vi "OutputRT.vi"(6 "Bias in":refnum<k21>, 7 "Monitor Task":refnum<k21>, 8 "rate":dbl=1000.0 format="%0.2f", 9 "MessageQueues":T1, 10 "Bias Voltage (mV)":string, 11 "TraceTime":dbl) -> ()   [LabVIEW 2024]
uses:
  MessageQueues.ctl
  <vilib>/httpClient/ClientHandle.ctl
  <vilib>/DAQmx/write.llb/DAQmx Write (Analog DBL 1Chan 1Samp).vi
  <vilib>/DAQmx/configure/timing.llb/DAQmx Timing (Sample Clock).vi
  <vilib>/DAQmx/miscellaneous.llb/DAQmx Fill In Error Info.vi
  <vilib>/httpClient/LabVIEWHTTPClient.lvlib
panel:
  in  "Sampling Rate: 3":dbl=5000.0
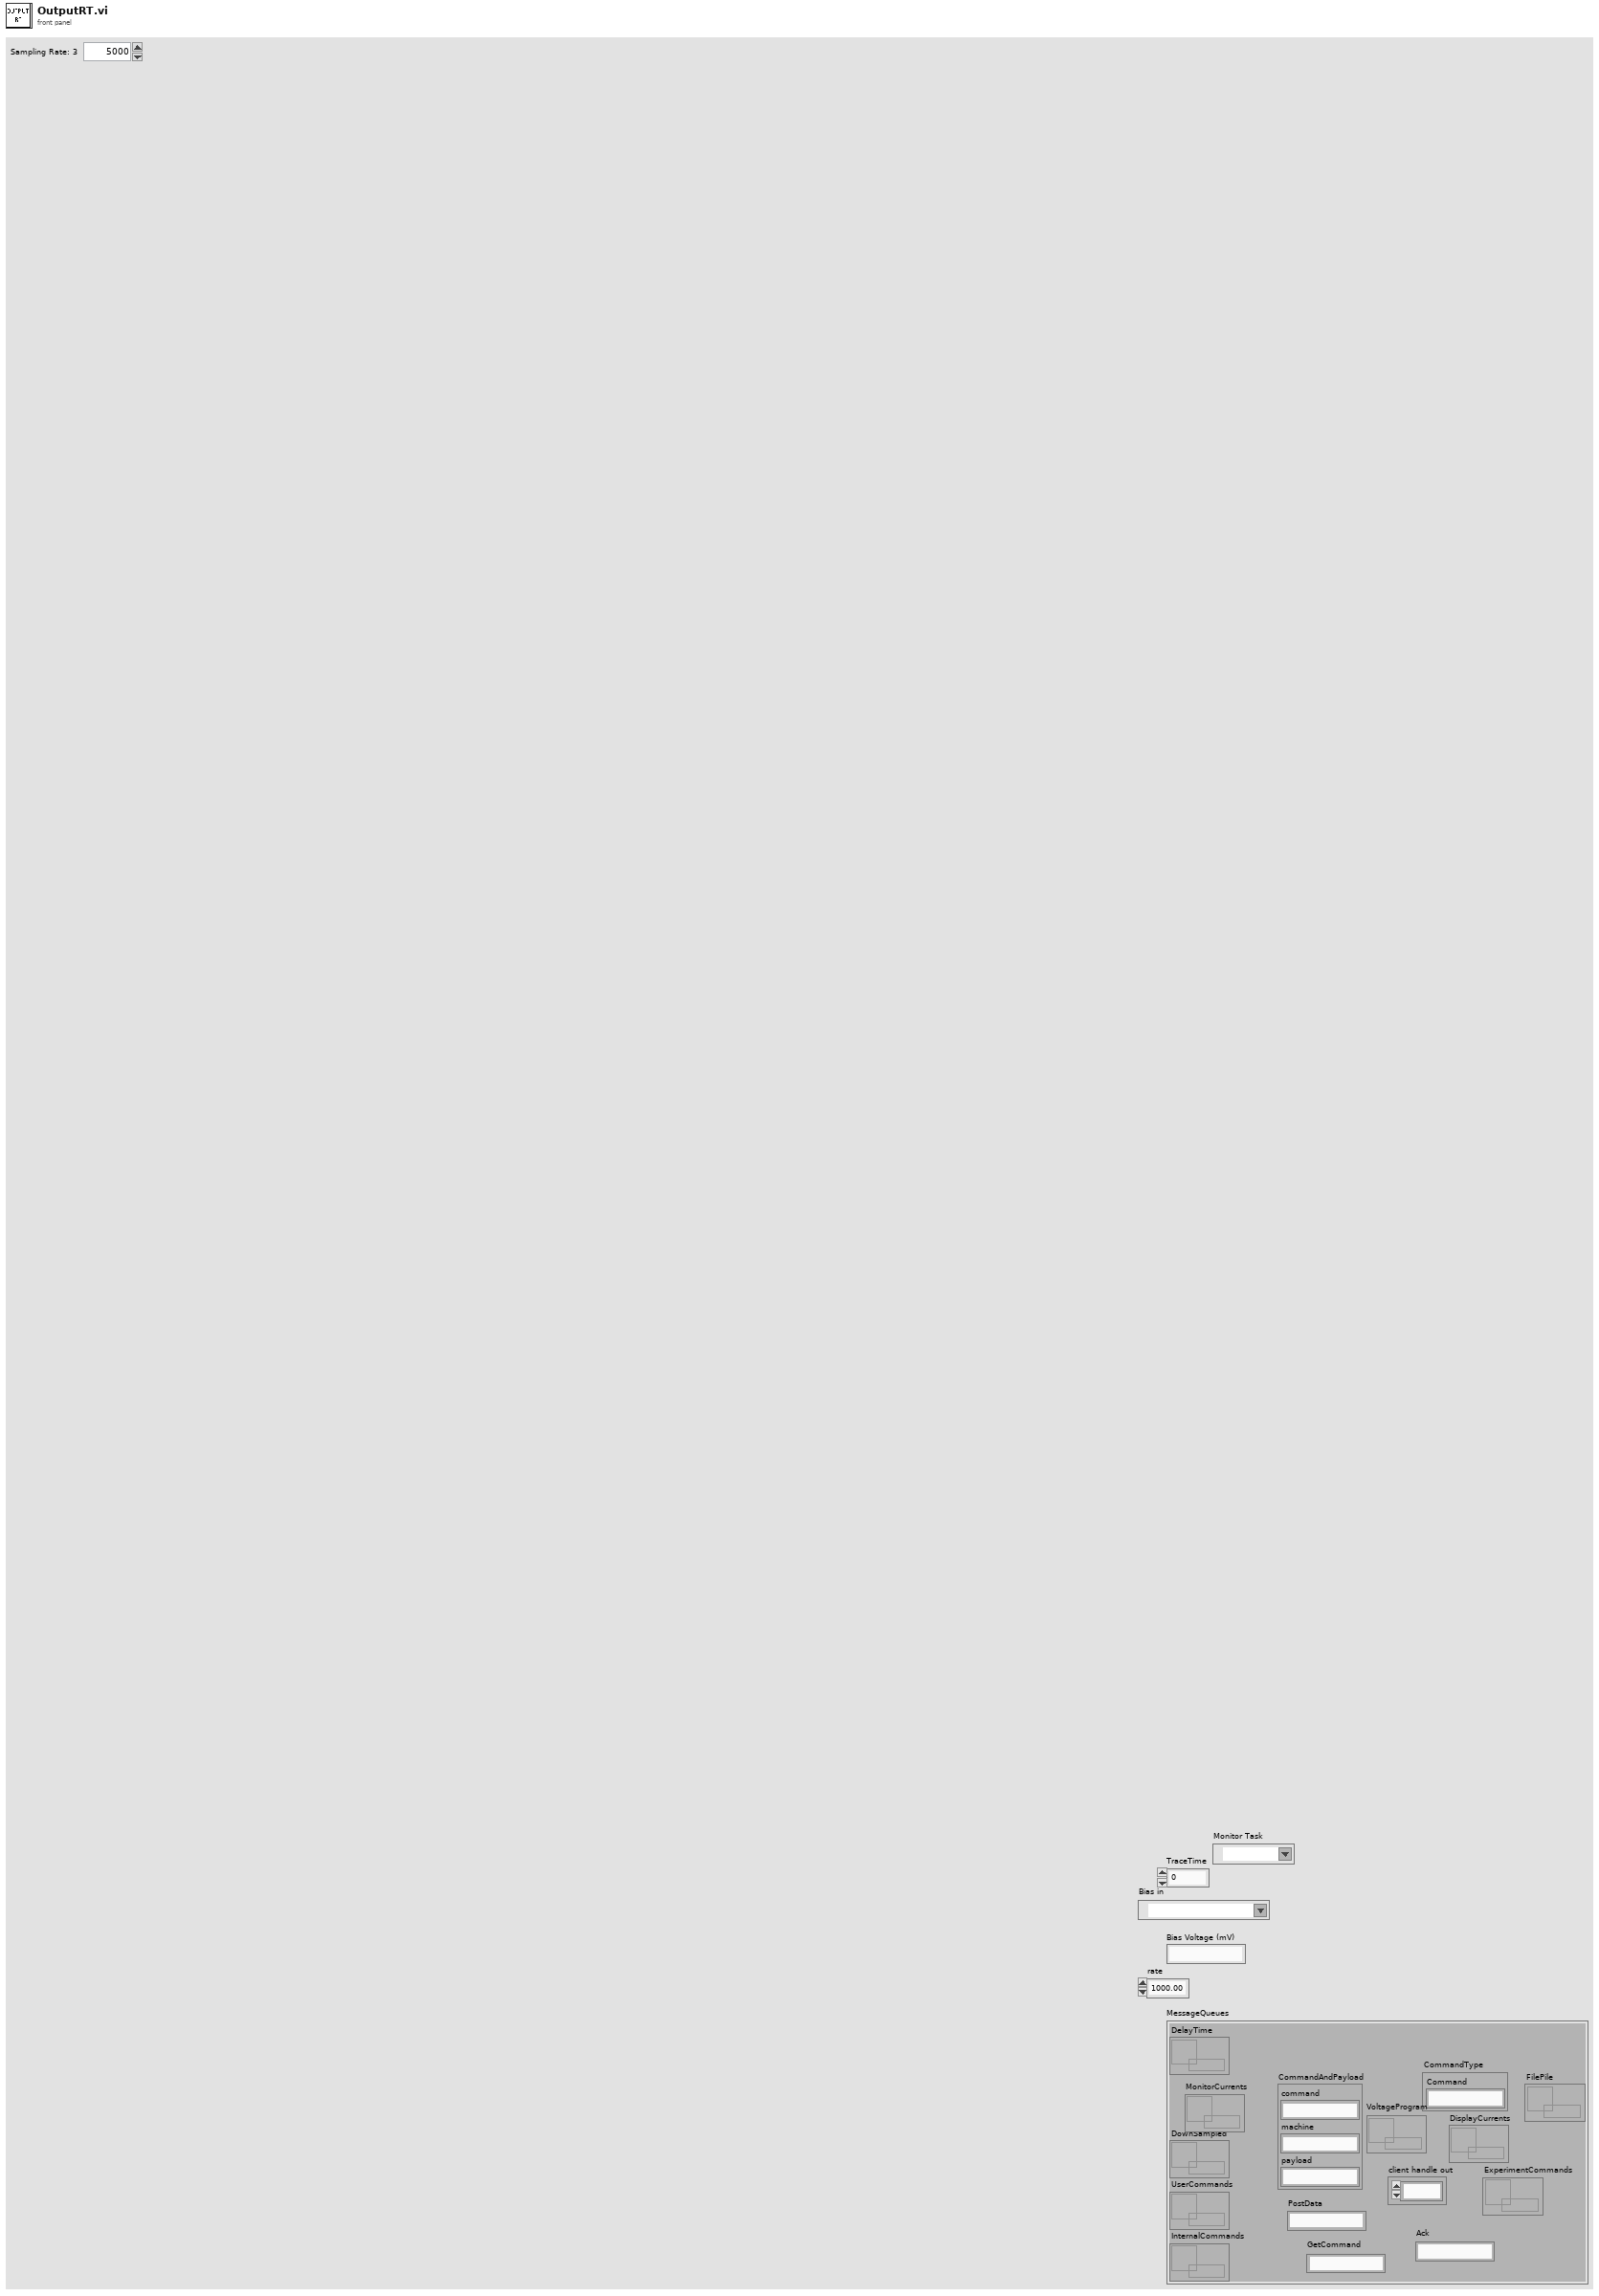
[diagram p1: front panel]
types:
  T1 = typedef "MessageQueues.ctl" = cluster{"DelayTime":refnum<queue>, "DownSampled":refnum<queue>, "UserCommands":refnum<queue>, "InternalCommands":refnum<queue>, "CommandType":cluster{"Command":string}, "CommandAndPayload":cluster{"command":string, "machine":string, "payload":string}, "client handle out":T2, "PostData":string, "GetCommand":string, "Ack":string, "VoltageProgram":refnum<queue>, "ExperimentCommands":refnum<queue>, "DisplayCurrents":refnum<queue>, "MonitorCurrents":refnum<queue>, "FilePile":refnum<queue>}
  T2 = typedef "LabVIEWHTTPClient.lvlib/ClientHandle.ctl" = refnum<k1>
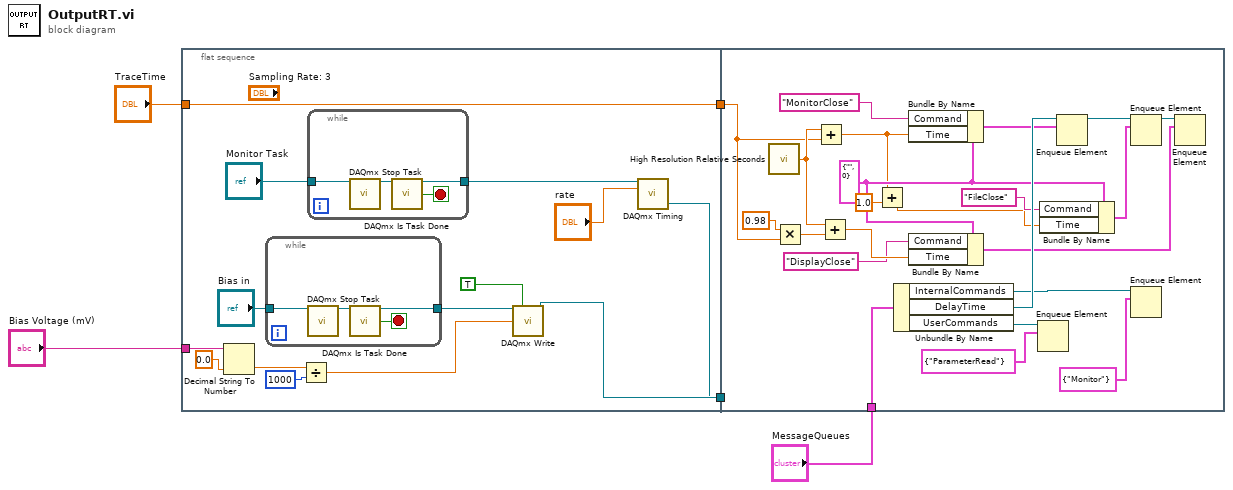
[diagram p0: block diagram]
diagram:
  n1 = flat-sequence {
    tunnel: [w20] -> w6
    tunnel: "TraceTime" -> [w20]
    tunnel: "Bias Voltage (mV)" -> [w18]
    tunnel: [w13] -> w5
    tunnel: [w11] -> w1
    tunnel: w6 -> [w33]
    tunnel: "MessageQueues" -> [w51]
    tunnel: w5 -> [_]
    tunnel: w1 -> [_]
    frame #0 {
      n2 = Decimal String To Number(string=w18, default (0L)=0.0) -> (number=w16:dbl)  [unwired: 1 in, 1 out]
      n3 = while {
        tunnel: "Bias in" -> [w28]
        tunnel: [w26] -> w9
        stop <- w25 stop-if-true
        n4 = call <vilib>:"DAQmx Stop Task.vi"("task/channels in"=w28) -> ("task out"=w27:refnum<k21>)  [unwired: 13 in, 1 out]
        n5 = call <vilib>:"DAQmx Is Task Done.vi"("task/channels in"=w27) -> ("task out"=w26:refnum<k21>, "task done?"=w25:bool)  [unwired: 12 in, 1 out]
      }
      n6 = Divide(x=w16, y=1000) -> (x/y=w15:dbl)
      n7 = while {
        tunnel: "Monitor Task" -> [w24]
        tunnel: [w22] -> w7
        stop <- w21 stop-if-true
        n8 = call <vilib>:"DAQmx Stop Task.vi"("task/channels in"=w24) -> ("task out"=w23:refnum<k21>)  [unwired: 13 in, 1 out]
        n9 = call <vilib>:"DAQmx Is Task Done.vi"("task/channels in"=w23) -> ("task out"=w22:refnum<k21>, "task done?"=w21:bool)  [unwired: 12 in, 1 out]
      }
      n10 = call-poly <vilib>:"DAQmx Write.vi"("task/channels in"=w9, "auto start"=TRUE, "data"=w15) -> ("task out"=w13:refnum<k21>)  [unwired: 10 in, 2 out]
      n11 = call-poly <vilib>:"DAQmx Timing.vi"("task/channels in"=w7, "rate"="rate") -> ("task out"=w11:refnum<k21>)  [unwired: 12 in, 1 out]
    }
    frame #1 {
      w36 = cluster{"Command":string, "Time":i32} {"Command"="", "Time"=0} ("element")
      n12 = call <vilib>:"High Resolution Relative Seconds.vi"() -> ("relative seconds"=w40:dbl)
      n13 = Multiply(x=0.98, y=w33) -> (x*y=w32:dbl)
      n14 = Add(x=w40, y=w33) -> (x+y=w31:dbl)
      n15 = Add(x=w40, y=w32) -> (x+y=w35:dbl)
      n16 = Add(x=w31, y=1.0) -> (x+y=w30:dbl)
      n17 = Unbundle By Name(w51) -> ("InternalCommands"=w45:refnum<queue>, "DelayTime"=w50:refnum<queue>, "UserCommands"=w46:refnum<queue>)
      n18 = Bundle By Name(cluster=w36, "Command"="MonitorClose", "Time"=w31) -> (w49:cluster{"Command":string, "Time":i32})
      n19 = Bundle By Name(cluster=w36, "Command"="DisplayClose", "Time"=w35) -> (w37:cluster{"Command":string, "Time":i32})
      n20 = Enqueue Element(queue=w46, element=cluster{"Command":string} {"Command"="ParameterRead"}) -> ()  [unwired: 2 in, 3 out]
      n21 = Bundle By Name(cluster=w36, "Command"="FileClose", "Time"=w30) -> (w43:cluster{"Command":string, "Time":i32})
      n22 = Enqueue Element(queue=w50, element=w49) -> (queue out=w39:refnum<queue>)  [unwired: 2 in, 2 out]
      n23 = Enqueue Element(queue=w39, element=w43) -> (queue out=w38:refnum<queue>)  [unwired: 2 in, 2 out]
      n24 = Enqueue Element(queue=w45, element=cluster{"Command":string} {"Command"="Monitor"}) -> ()  [unwired: 2 in, 3 out]
      n25 = Enqueue Element(queue=w38, element=w37) -> ()  [unwired: 2 in, 3 out]
    }
  }
